vi "Init Movables.vi"(11 "Game Board in":refnum<class "Game Board.lvclass">) -> (3 "Game Board out":refnum<class "Game Board.lvclass">)   [LabVIEW 2021, in "Game Board.lvclass"]
doc: "MIT Licence\nCopyright (c) 2024 David Grollier"
uses:
  Game Board.lvclass
  Game Board.lvclass/Game Board.ctl
  Type Def/Coordinates.ctl
  Game Board Component/Movable/Ball/Ball.lvclass
  C:/Users/David/Documents/GameSoccerSpace/Source/Game Componants/Game Board Component/Movable/Movable.lvclass
  Game Board Component/Movable/Flying Saucer/Flying Saucer.lvclass
  Game Board Component/Movable/Movable.lvclass
  C:/Users/David/Documents/GameSoccerSpace/Source/Game Componants/Game Board Component/Game Board Component.lvclass
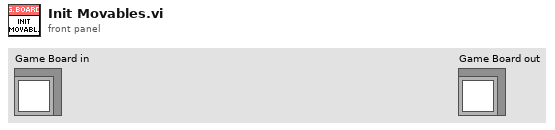
[diagram p1: front panel]
types:
  T1 = typedef "LVBoundsTypeDef.ctl" = cluster{"Width":u32, "Height":u32}
  T2 = typedef "Coordinates.ctl" = cluster{"x":dbl, "y":dbl}
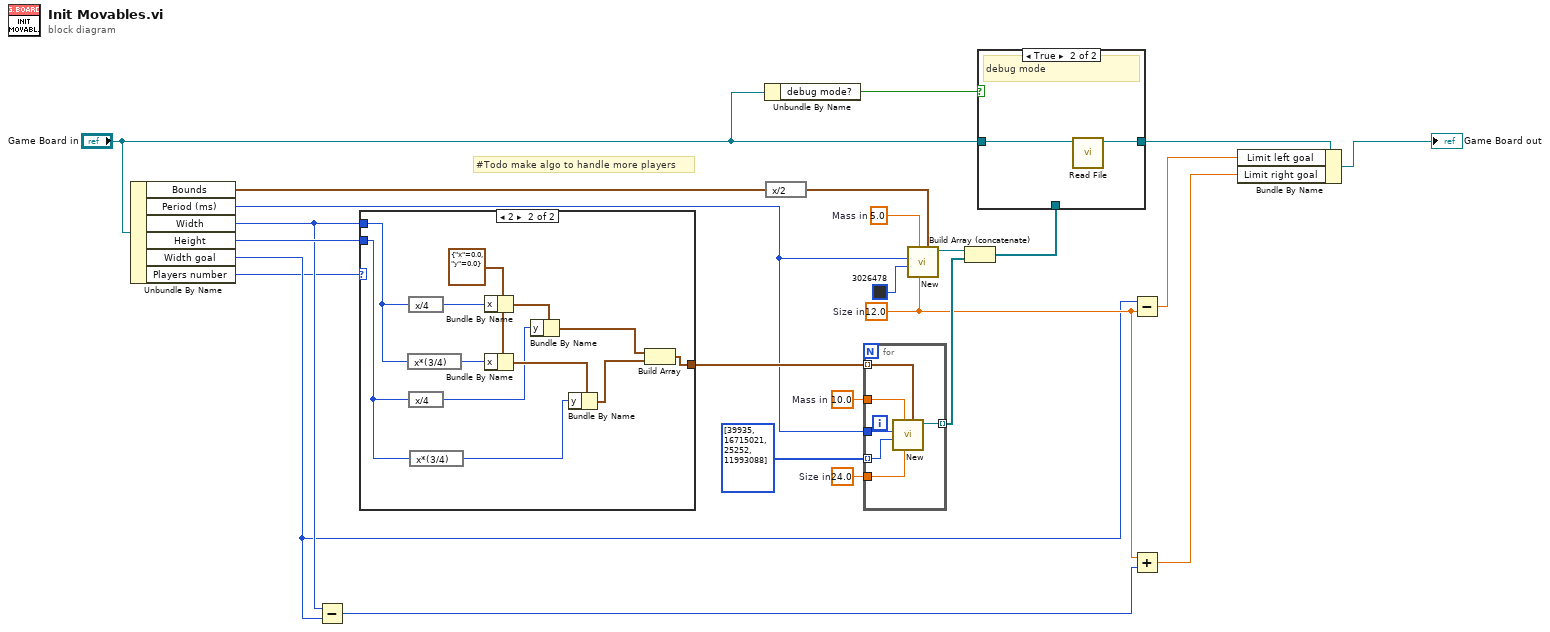
[diagram p0: block diagram]
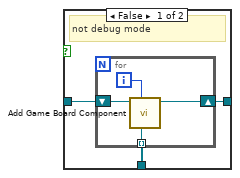
[diagram p2: hidden frame]
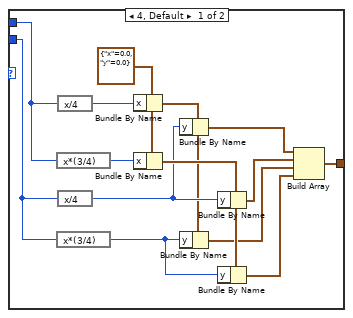
[diagram p3: hidden frame]
diagram:
  w20 = 10.0  # Mass in
  w21 = 24.0  # Size in
  w24 = 5.0  # Mass in
  w8 = 12.0  # Size in
  # "#Todo make algo to handle more players"
  n1 = Unbundle By Name("Game Board in") -> ("Bounds"=w15:T1, "Period (ms)"=w4:i64, "Width"=w7:u32, "Height"=w13:u32, "Width goal"=w6:u16, "Players number"=w3:u8)
  n2 = Subtract(x=w7, y=w6) -> (x-y=w5:u32)
  n3 = case shown="2" w3 {
    tunnel: w13 -> [w37 w40]
    tunnel: [w29 w45] -> w12
    tunnel: w7 -> [w27 w43]
    frame 4, Default {
      w36 = T2 {"x"=0.0, "y"=0.0} ("Coordinates in")
      n4 = expression code="x*(3/4)"(w27) -> (w32:u32)
      n5 = expression code="x*(3/4)"(w37) -> (w33:u32)
      n6 = expression code="x/4"(w27) -> (w38:u32)
      n7 = expression code="x/4"(w37) -> (w34:u32)
      n8 = Bundle By Name(cluster=w36, "x"=w38) -> (w28:T2)
      n9 = Bundle By Name(cluster=w36, "x"=w32) -> (w35:T2)
      n10 = Bundle By Name(cluster=w28, "y"=w34) -> (w31:T2)
      n11 = Bundle By Name(cluster=w28, "y"=w33) -> (w25:T2)
      n12 = Bundle By Name(cluster=w35, "y"=w34) -> (w26:T2)
      n13 = Bundle By Name(cluster=w35, "y"=w33) -> (w30:T2)
      n14 = Build Array(w31, w26, w25, w30) -> (w29:T2[])
    }
    frame 2 {
      w49 = T2 {"x"=0.0, "y"=0.0} ("Coordinates in")
      n15 = expression code="x*(3/4)"(w43) -> (w47:u32)
      n16 = expression code="x/4"(w43) -> (w50:u32)
      n17 = expression code="x/4"(w40) -> (w41:u32)
      n18 = expression code="x*(3/4)"(w40) -> (w39:u32)
      n19 = Bundle By Name(cluster=w49, "x"=w50) -> (w44:T2)
      n20 = Bundle By Name(cluster=w49, "x"=w47) -> (w48:T2)
      n21 = Bundle By Name(cluster=w44, "y"=w41) -> (w46:T2)
      n22 = Bundle By Name(cluster=w48, "y"=w39) -> (w42:T2)
      n23 = Build Array(w46, w42) -> (w45:T2[])
    }
  }
  n24 = Unbundle By Name("Game Board in") -> ("debug mode?"=w1:bool)
  n25 = expression code="x/2"(w15) -> (w14:T1)
  n26 = for {
    tunnel: [w56] -> w23 mode=indexing
    tunnel: w21 -> [w55]
    tunnel: w20 -> [w54]
    tunnel: u32[] [39935, 16715021, 25252, 11993088] ("color in") -> [w53] mode=indexing
    tunnel: w12 -> [w52] mode=indexing
    tunnel: w4 -> [w51]
    n27 = call "New.vi"("Coordinates in"=w52, "Size in"=w55, "Mass in"=w54, "color in"=w53, "Period (ms) in"=w51) -> ("Flying Saucer out"=w56:refnum<class "Flying Saucer.lvclass">)  [unwired: 6 in]
  }
  n28 = call "New.vi"("Coordinates in"=w14, "Size in"=w8, "Mass in"=w24, "color in"=u32 3026478, "Period (ms) in"=w4) -> ("Ball out"=w19:refnum<class "Ball.lvclass">)  [unwired: 6 in]
  n29 = Build Array (concatenate)(w19, w23) -> (w18:refnum<class "Movable.lvclass">[])
  n30 = case shown="True" w1 {
    tunnel: w18 -> [w59 _]
    tunnel: [w58 w64] -> w16
    tunnel: "Game Board in" -> [w57 w65]
    frame False {
      # "not debug mode"
      n31 = for {
        shift-right: [w62] -> w58
        shift-left: w57 -> [w63]
        tunnel: w59 -> [w61] mode=indexing
        i -> [w60]
        n32 = call "Add Game Board Component.vi"("Game Board Component in"=w61, "Index in"=w60, "Game Board in"=w63) -> ("Game Board out"=w62:refnum<class "Game Board.lvclass">)  [unwired: 8 in]
      }
    }
    frame True {
      # "debug mode"
      n33 = call "Read File.vi"("Game Board in"=w65) -> ("Game Board out"=w64:refnum<class "Game Board.lvclass">)  [unwired: 9 in, 1 out]
    }
  }
  n34 = Subtract(x=w6, y=w8) -> (x-y=w10:dbl)
  n35 = Add(x=w8, y=w5) -> (x+y=w9:dbl)
  n36 = Bundle By Name(cluster=w16, "Limit left goal"=w10, "Limit right goal"=w9) -> (→"Game Board out":refnum<class "Game Board.lvclass">)
